vi "OBIS Set Power.vi"() -> ()   [LabVIEW 8.6]
uses:
  <vilib>/Instr/_visa.llb/VISA Configure Serial Port (Instr).vi
panel:
  in  "Set":bool
  out "Diode Temp":dbl
  out "Diode Current":dbl
  out "Laser Power":dbl
  in  "stop":bool
  in  "Set Laser Power":dbl(slide) scale format="%.1f"
  in  "VISA resource name":refnum<visa-resource-name>
  # "mW"
  # "mW"
  # "mA"
  # "°C"
  # "This VI can be used to control the power level of the laser.  Select the appropriate VISA resouce name (COM port number) for the laser and run this VI.  It will read the current laser power and allow that to be adjusted.  The measured laser power (from the internal photodiode) is reported along with the diode current and diode temperature.  After setting a new laser power level, press the SET button to accept the changes."
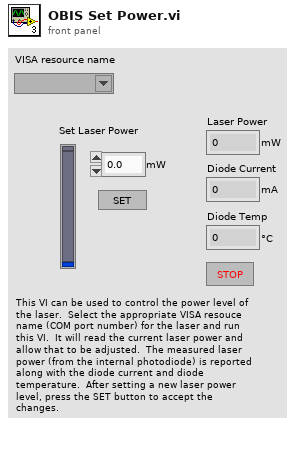
[diagram p1: front panel]
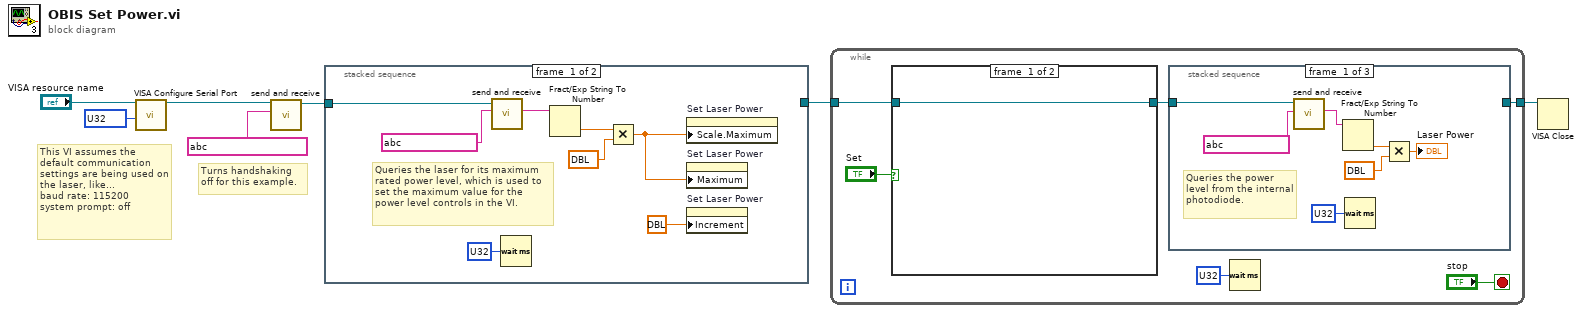
[diagram p0: block diagram]
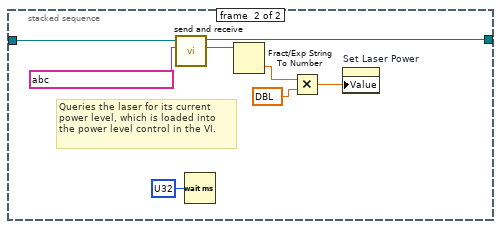
[diagram p2: hidden frame]
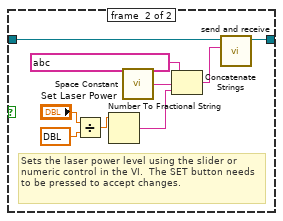
[diagram p3: hidden frame]
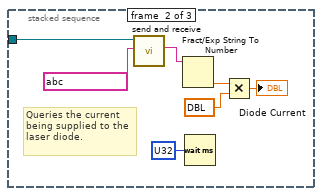
[diagram p4: hidden frame]
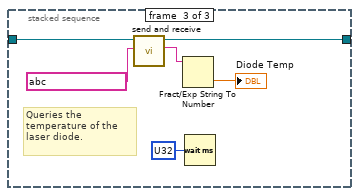
[diagram p5: hidden frame]
diagram:
  # "Turns handshaking\noff for this example."
  # "This VI assumes the default communication settings are being used on the laser, like...\nbaud rate: 115200\nsystem prompt: off"
  n1 = call-poly "VISA Configure Serial Port"("VISA resource name"="VISA resource name", "baud rate (9600)"=u32 ?) -> ("VISA resource name out"=w2:refnum<visa-resource-name>)  [unwired: 12 in, 1 out]
  n2 = call "send and receive.vi"("write to laser"=string ?, "VISA resource name"=w2) -> ("VISA resource name out"=w1:refnum<visa-resource-name>)  [unwired: 8 in, 1 out]
  n3 = stacked-sequence {
    tunnel: [_ w21] -> w7
    tunnel: w1 -> [w9 w16]
    frame #0 {
      # "Queries the laser for its maximum rated power level, which is used to set the maximum value for the power level controls in the VI."
      n4 = call "send and receive.vi"("write to laser"=string ?, "VISA resource name"=w9) -> ("read from laser"=w14:string)  [unwired: 8 in, 1 out]
      n5 = Wait (ms)(milliseconds to wait=u32 ?) -> ()  [unwired: 1 out]
      n6 = Fract/Exp String To Number(string=w14) -> (number=w11:dbl)  [unwired: 3 in, 1 out]
      n7 = Multiply(x=w11, y=dbl ?) -> (x*y=w12:dbl)
      n8 = property on="Set Laser Power" class="Slide (strict)"("Scale.Maximum"=w12) -> ()  [unwired: 2 in, 2 out]
      n9 = property on="Set Laser Power" class="Slide (strict)"("Maximum"=w12) -> ()  [unwired: 2 in, 2 out]
      n10 = property on="Set Laser Power" class="Slide (strict)"("Increment"=dbl ? ("y")) -> ()  [unwired: 2 in, 2 out]
    }
    frame #1 {
      # "Queries the laser for its current power level, which is loaded into the power level control in the VI."
      n11 = call "send and receive.vi"("write to laser"=string ?, "VISA resource name"=w16) -> ("read from laser"=w22:string, "VISA resource name out"=w21:refnum<visa-resource-name>)  [unwired: 8 in]
      n12 = Wait (ms)(milliseconds to wait=u32 ?) -> ()  [unwired: 1 out]
      n13 = Fract/Exp String To Number(string=w22) -> (number=w20:dbl)  [unwired: 3 in, 1 out]
      n14 = Multiply(x=w20, y=dbl ?) -> (x*y=w17:dbl)
      n15 = property on="Set Laser Power" class="Slide (strict)"("Value"=w17) -> ()  [unwired: 2 in, 2 out]
    }
  }
  n16 = while {
    tunnel: w7 -> [w25]
    tunnel: [w28] -> w4
    stop <- "stop" stop-if-true
    n17 = case shown="True" "Set" {
      tunnel: w25 -> [w30 w32]
      tunnel: [w30 w31] -> w24
      frame #0 {
      }
      frame #1 {
        # "Sets the laser power level using the slider or numeric control in the VI.  The SET button needs to be pressed to accept changes."
        n18 = Divide(x="Set Laser Power", y=dbl ?) -> (x/y=w33:dbl)
        n19 = Number To Fractional String(number=w33) -> (F-format string=w37:string)  [unwired: 3 in]
        n20 = call <vilib>:"Space Constant.vi"() -> ("String"=w38:string)
        n21 = Concatenate Strings(string ?, w38, w37) -> (w36:string)
        n22 = call "send and receive.vi"("write to laser"=w36, "VISA resource name"=w32) -> ("VISA resource name out"=w31:refnum<visa-resource-name>)  [unwired: 8 in, 1 out]
      }
    }
    n23 = stacked-sequence {
      tunnel: w24 -> [w44 w50 w58]
      tunnel: [_ _ w56] -> w28
      frame #0 {
        # "Queries the power level from the internal photodiode."
        n24 = call "send and receive.vi"("write to laser"=string ?, "VISA resource name"=w44) -> ("read from laser"=w46:string)  [unwired: 8 in, 1 out]
        n25 = Fract/Exp String To Number(string=w46) -> (number=w45:dbl)  [unwired: 3 in, 1 out]
        n26 = Wait (ms)(milliseconds to wait=u32 ?) -> ()  [unwired: 1 out]
        n27 = Multiply(x=w45, y=dbl ?) -> (x*y=→"Laser Power":dbl)
      }
      frame #1 {
        # "Queries the current being supplied to the laser diode."
        n28 = call "send and receive.vi"("write to laser"=string ?, "VISA resource name"=w50) -> ("read from laser"=w52:string)  [unwired: 8 in, 1 out]
        n29 = Fract/Exp String To Number(string=w52) -> (number=w51:dbl)  [unwired: 3 in, 1 out]
        n30 = Wait (ms)(milliseconds to wait=u32 ?) -> ()  [unwired: 1 out]
        n31 = Multiply(x=w51, y=dbl ?) -> (x*y=→"Diode Current":dbl)
      }
      frame #2 {
        # "Queries the temperature of the laser diode."
        n32 = call "send and receive.vi"("write to laser"=string ?, "VISA resource name"=w58) -> ("read from laser"=w59:string, "VISA resource name out"=w56:refnum<visa-resource-name>)  [unwired: 8 in]
        n33 = Fract/Exp String To Number(string=w59) -> (number=→"Diode Temp":dbl)  [unwired: 3 in, 1 out]
        n34 = Wait (ms)(milliseconds to wait=u32 ?) -> ()  [unwired: 1 out]
      }
    }
    n35 = Wait (ms)(milliseconds to wait=u32 ?) -> ()  [unwired: 1 out]
  }
  n36 = VISA Close(VISA resource name=w4) -> ()  [unwired: 1 in, 1 out]
